vi "fir_test3.vi"() -> ()   [LabVIEW 2013]
uses:
  <vilib>/measure/maspectr.llb/Power Spectrum and PSD Export Mode.ctl
  <vilib>/measure/maspectr.llb/FFT Power Spectrum and PSD for 1 Chan.vi
  <vilib>/measure/NI_MABase.lvlib
  <vilib>/measure/NI_MAPro.lvlib
panel:
  out "Waveform Graph out":dbl[](graph)
  out "Power spectrum in":cluster{"f0":dbl, "df":dbl, "magnitude":dbl[]}(graph)
  out "Power spectrum":cluster{"f0":dbl, "df":dbl, "magnitude":dbl[]}(graph)
  out "Waveform Graph":dbl[](graph)
  out "# of Iterations":i32
  out "# of samples":i32
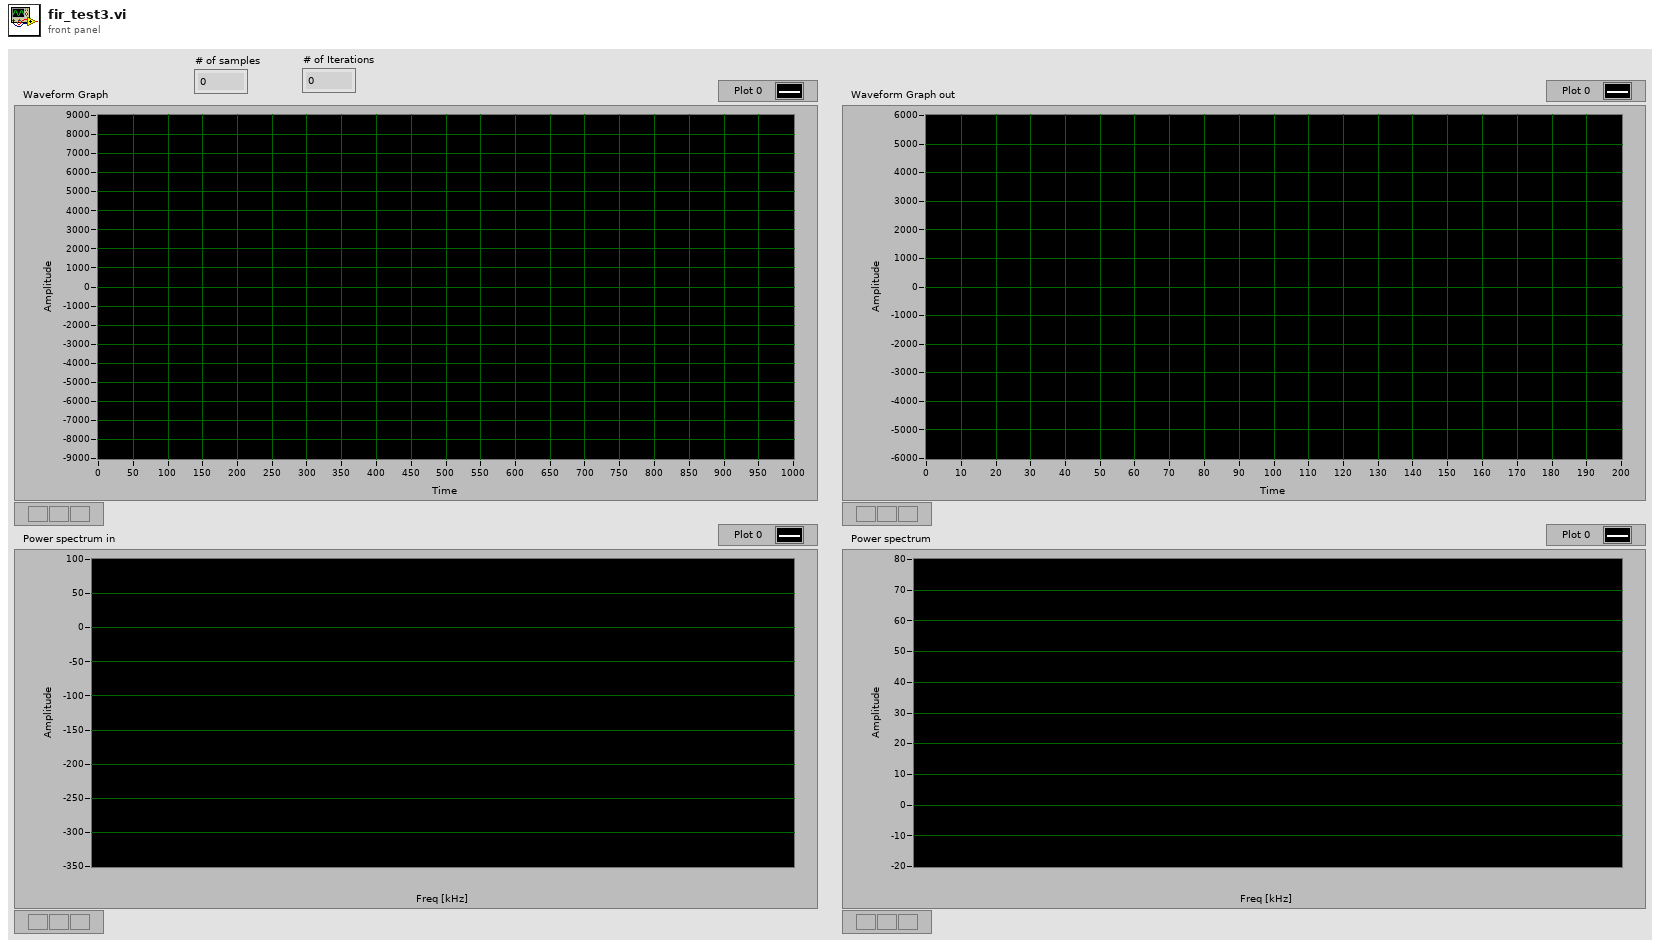
[diagram p1: front panel]
types:
  T1 = typedef "NI_MAPro.lvlib/Power Spectrum and PSD Export Mode.ctl" = u16
  T2 = cluster{"frequency":dbl, "amplitude":dbl, "phase":dbl}[]
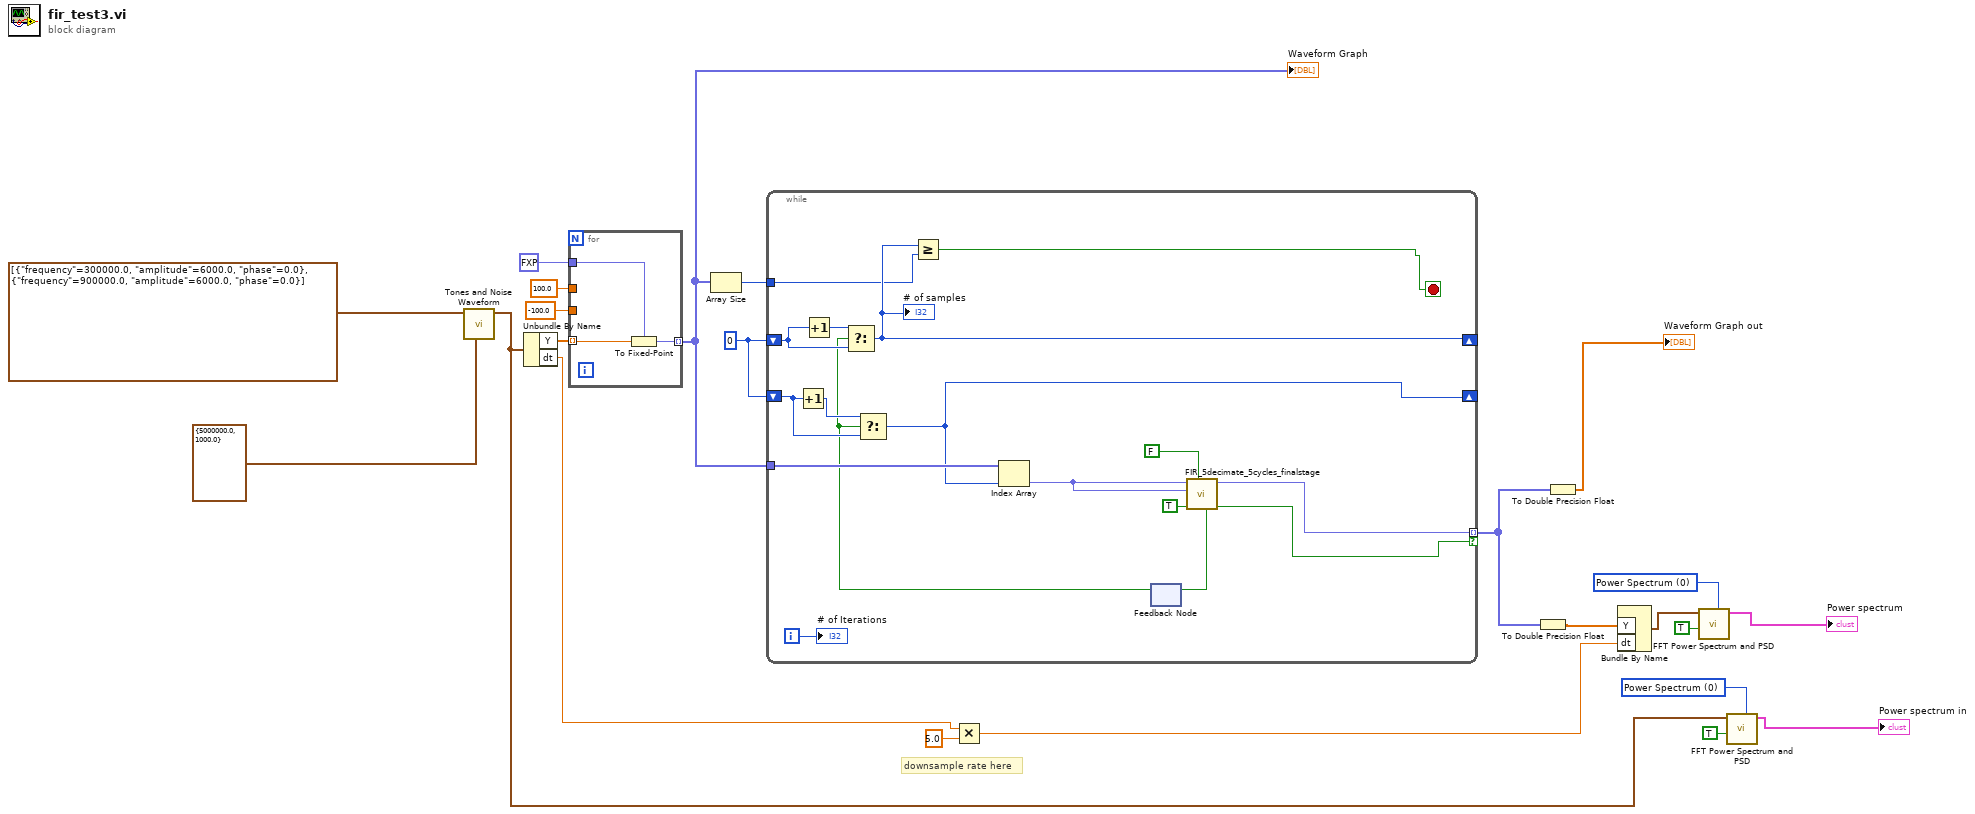
[diagram p0: block diagram]
diagram:
  w8 = T1 0 items=["Power Spectrum", "Power Spectral Density"] ("export mode")
  w17 = T1 0 items=["Power Spectrum", "Power Spectral Density"] ("export mode")
  w19 = 0 ("samples")
  # "downsample rate here"
  n1 = call <vilib>:"Tones and Noise Waveform.vi"("sampling info"=cluster{"Fs":dbl, "#s":dbl} {"Fs"=5000000.0, "#s"=1000.0}, "tones"=T2 [{"frequency"=300000.0, "amplitude"=6000.0, "phase"=0.0}, {"frequency"=900000.0, "amplitude"=6000.0, "phase"=0.0}]) -> ("signal out"=w7:waveform(dbl))  [unwired: 8 in, 1 out]
  n2 = Unbundle By Name(w7) -> ("Y"=w15:dbl[], "dt"=w14:dbl)
  n3 = for {
    tunnel: w15 -> [w24] mode=indexing
    tunnel: fxp<+/-,16,14> 0.0 ("fixed-point type") -> [w26]
    tunnel: [w25] -> w3 mode=indexing
    tunnel: 100.0 -> [_]
    tunnel: -100.0 -> [_]
    n4 = To Fixed-Point(fixed-point type=w26, number=w24) -> (fixed-point=w25:fxp<+/-,16,14>)
  }
  "Waveform Graph" <- w3
  n5 = Array Size(array=w3) -> (size(s)=w20:i32)
  n6 = while {
    tunnel: w3 -> [w43]
    shift-right: [w35] -> _
    shift-left: w19 -> [w41]
    shift-right: [w38] -> _
    shift-left: w19 -> [w39]
    tunnel: [w29] -> w5 mode=indexing if=w28
    tunnel: w20 -> [w36]
    i -> [w34]
    stop <- w37 stop-if-true
    n7 = Increment(x=w41) -> (x+1=w42:i32)
    n8 = Increment(x=w39) -> (x+1=w40:i32)
    n9 = feedback #1() -> (w27:bool)  [unwired: 1 in]
    n10 = Select(t=w40, s=w27, f=w39) -> (s? t:f=w38:i32)
    "# of samples" <- w38
    n11 = Select(t=w42, s=w27, f=w41) -> (s? t:f=w35:i32)
    n12 = Greater Or Equal?(x=w38, y=w36) -> (x >= y?=w37:bool)
    n13 = Index Array(array=w43, index=w35) -> (element=w33:fxp<+/-,16,14>)
    n14 = call "FIR_5decimate_5cycles_finalstage.vi"("reset"=FALSE, "valid in"=TRUE, "Q in"=w33, "I in"=w33) -> ("valid out"=w28:bool, "I out"=w29:fxp<+/-,16,14>, "ready for input"=w32:bool)  [unwired: 4 in, 1 out]
    n15 = feedback-in #1(w32) -> ()
    "# of Iterations" <- w34
  }
  n16 = Multiply(x=w14, y=5.0) -> (x*y=w12:dbl)
  n17 = To Double Precision Float(number=w5) -> (double precision float=w10:dbl[])
  n18 = To Double Precision Float(number=w5) -> (double precision float=→"Waveform Graph out":dbl[])
  n19 = Bundle By Name("Y"=w10, "dt"=w12) -> (w18:waveform(dbl))  [unwired: 1 in]
  n20 = call-poly <vilib>:"FFT Power Spectrum and PSD.vi"("export mode"=w17, "dB On (F)"=TRUE, "time signal"=w18) -> ("Power Spectrum / PSD"=→"Power spectrum":cluster{"f0":dbl, "df":dbl, "magnitude":dbl[]})  [unwired: 5 in, 3 out]
  n21 = call-poly <vilib>:"FFT Power Spectrum and PSD.vi"("export mode"=w8, "dB On (F)"=TRUE, "time signal"=w7) -> ("Power Spectrum / PSD"=→"Power spectrum in":cluster{"f0":dbl, "df":dbl, "magnitude":dbl[]})  [unwired: 5 in, 3 out]
